vi "demo.vi"() -> ()   [LabVIEW 2013]
panel:
  out "No Compression":bool
  out "Bad Compression":bool
  out "XY Graph":cluster{dbl[], dbl[]}(graph)
  out "Countdown":dbl
  in  "Start Delay (s)":u32=1 max=10 step=1
  in  "Show Debug":bool
  out "Compression Depth":dbl(slide) scale=0.0..6.0
  out "Compression Rate":i16(slide) scale=0.0..200.0
  out "Too Deep":bool
  out "Good  2":bool
  out "Too Shallow":bool
  out "Too Slow":bool
  out "Good":bool
  out "Too Fast":bool
  in  "Sample Period (s)":i8(knob)=2 min=2 max=10 step=1 scale=0.0..10.0 scale format="%#1_6g"
  in  "Stop Button":bool
  in  "Start/Stop Training":bool
  # "SMART Anne"
  # "A low-cost, lightweight CPR mannequin outfitted with inertial sensors that provide real-time feedback"
  # "Controls"
  # "Feedback"
  # "Debug"
  # "Compression Rate"
  # "Too Slow"
  # "Too Fast"
  # "Compression Depth"
  # "+"
  # "-"
  # "Too Shallow"
  # "Too Deep"
  # "Chris Williams          Last Updated: Apr 13, 2017"
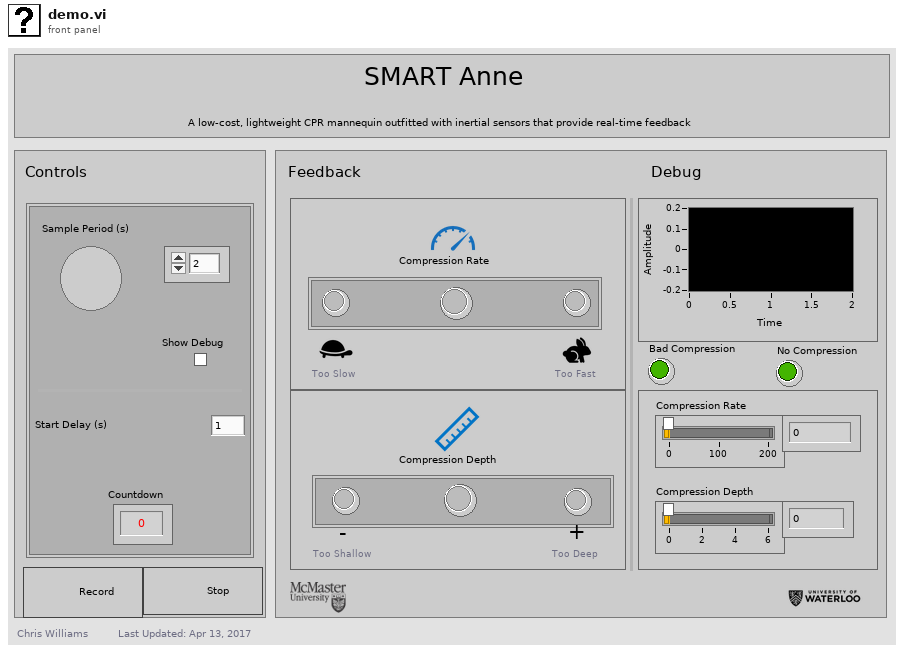
[diagram p1: front panel]
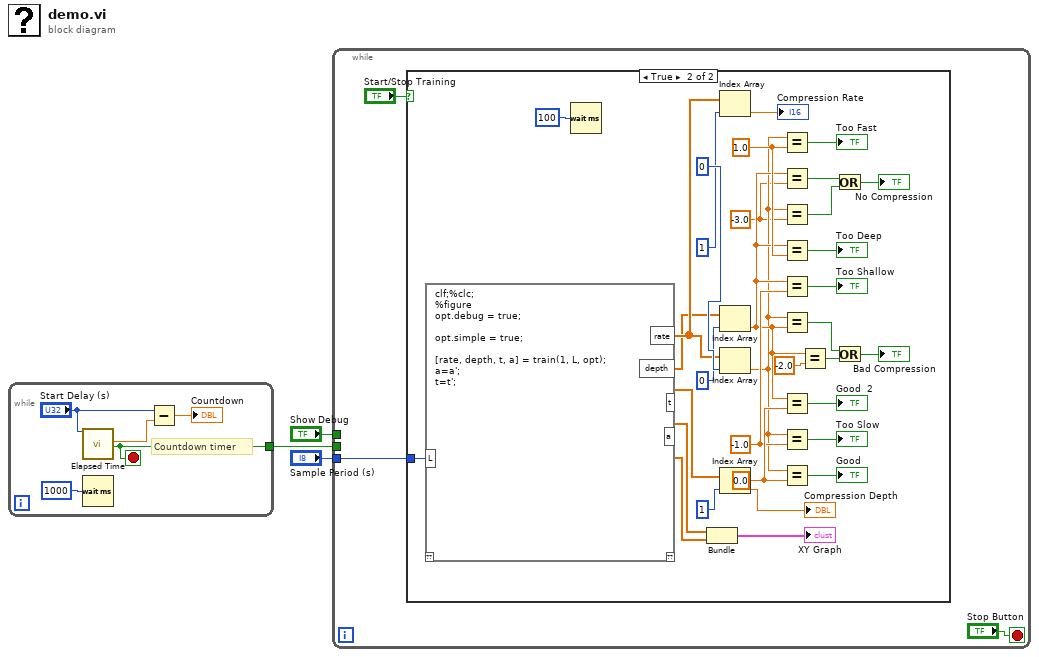
[diagram p0: block diagram]
diagram:
  n1 = while {
    tunnel: [w6] -> w3
    stop <- w6 stop-if-true
    # "Countdown timer"
    n2 = call "Elapsed Time"("Time Target (s)"="Start Delay (s)") -> ("Elapsed Time (s)"=w8:dbl, "Time has Elapsed"=w6:bool)  [unwired: 11 in, 6 out]
    n3 = Wait (ms)(milliseconds to wait=u32 1000) -> ()  [unwired: 1 out]
    n4 = Subtract(x="Start Delay (s)", y=w8) -> (x-y=→"Countdown":dbl)
  }
  n5 = while {
    tunnel: w3 -> [_]
    tunnel: "Sample Period (s)" -> [w9]
    tunnel: "Show Debug" -> [_]
    stop <- "Stop Button" stop-if-true
    n6 = case shown="True" "Start/Stop Training" {
      tunnel: w9 -> [_ w29]
      frame False {
      }
      frame True {
        w13 = -3.0 ("y")
        w23 = 0.0 ("y")
        w21 = 1.0 ("y")
        w22 = -1.0 ("y")
        n7 = script code="clf;%clc;\n%figure\nopt.debug = true;\n\nopt.simple = true;\n\n[rate, depth, t, a] = train(1, L, opt);\na=a';\nt=t';"("L"=w29) -> ("rate"=w35:dbl[], "depth"=w33:dbl[], "t"=w26:dbl[], "a"=w25:dbl[])  [unwired: 1 in, 1 out]
        n8 = Wait (ms)(milliseconds to wait=u32 100) -> ()  [unwired: 1 out]
        n9 = Bundle(w26, w25) -> (→"XY Graph":cluster{dbl[], dbl[]})  [unwired: 1 in]
        n10 = Index Array(array=w35, index=1) -> (element=→"Compression Rate":dbl)
        n11 = Index Array(array=w33, index=0) -> (element=w17:dbl)
        n12 = Index Array(array=w35, index=0) -> (element=w16:dbl)
        n13 = Index Array(array=w33, index=1) -> (element=→"Compression Depth":dbl)
        n14 = Equal?(x=w16, y=w21) -> (x = y?=→"Too Fast":bool)
        n15 = Equal?(x=w17, y=w13) -> (x = y?=w15:bool)
        n16 = Equal?(x=w16, y=w13) -> (x = y?=w14:bool)
        n17 = Equal?(x=w17, y=w21) -> (x = y?=→"Too Deep":bool)
        n18 = Equal?(x=w17, y=w22) -> (x = y?=→"Too Shallow":bool)
        n19 = Equal?(x=w16, y=w17) -> (x = y?=w19:bool)
        n20 = Equal?(x=w17, y=w23) -> (x = y?=→"Good  2":bool)
        n21 = Equal?(x=w16, y=w22) -> (x = y?=→"Too Slow":bool)
        n22 = Equal?(x=w16, y=w23) -> (x = y?=→"Good":bool)
        n23 = Equal?(x=w17, y=-2.0) -> (x = y?=w20:bool)
        n24 = Or(x=w15, y=w14) -> (x .or. y?=→"No Compression":bool)
        n25 = Or(x=w19, y=w20) -> (x .or. y?=→"Bad Compression":bool)
      }
    }
  }
